vi "test_PinGroup_ReserveSessions_GroupMappingsContainsPinGroup.vi"() -> (6 "pass":bool, 8 "result":string, 15 "error out":errorcluster)   [LabVIEW 2020, in "MeasurementServerTests.lvlib" / "Session Reservation Tests.lvlib"]
uses:
  Session Reservation Tests.lvlib
  gRPC/Generated APIs/ni/measurementlink/sessionmanagement/v1/RPC Messages/ni_measurementlink_PinMapContext.ctl
  Runtime/APIs/Session Management V1/Session Reservation/Group Mapping.ctl
  Runtime/APIs/Session Management V1/Session Reservation/Session Reservation.lvclass/Session Reservation.ctl
  ab61e54b-70f9-4719-86d2-c3025959eeb5.vi
  3347d1b6-dca7-4e1a-9ca0-c9ec2f5aba95.vi
  Runtime/APIs/Session Management V1/Session Reservation/Merge Invalid DVR Error.vi
  Runtime/APIs/Session Management V1/Session Reservation/Is DVR Valid.vi
  Runtime/Measurements/Helpers/Error Strings Global Internal.vi
  <vilib>/Utility/error.llb/Error Cluster From Error Code.vi
  <vilib>/JDP Science/JSONtext/Variant to JSON Text.vi
  <vilib>/JDP Science/JSONtext/LVClass Serializer/JSONtext LVClass Serializer.lvclass
  gRPC/Generated APIs/ni/measurementlink/sessionmanagement/v1/ni.measurementlink.sessionmanagement.v1.api.lvlib
  MeasurementServerTests.lvlib
  Runtime/APIs/Session Management V1/Session Reservation/Session Reservation.lvclass
panel:
  # "Test assumes discovery service, pin map service, and session management service have already been started."
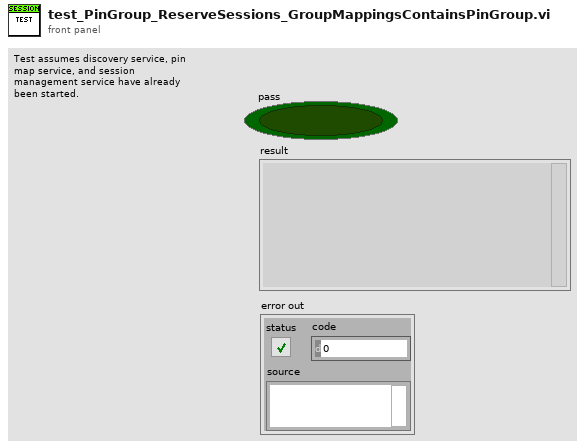
[diagram p1: front panel]
types:
  T1 = typedef "Plug-In SDK Session Management V1 API.lvlib/Session Reservation.lvclass/Group Mapping.ctl" = map{string, string[]}
  T2 = typedef "ni.measurementlink.sessionmanagement.v1.api.lvlib/ni_measurementlink_PinMapContext.ctl" = cluster{"pin_map_id":string, "sites":i32[]}
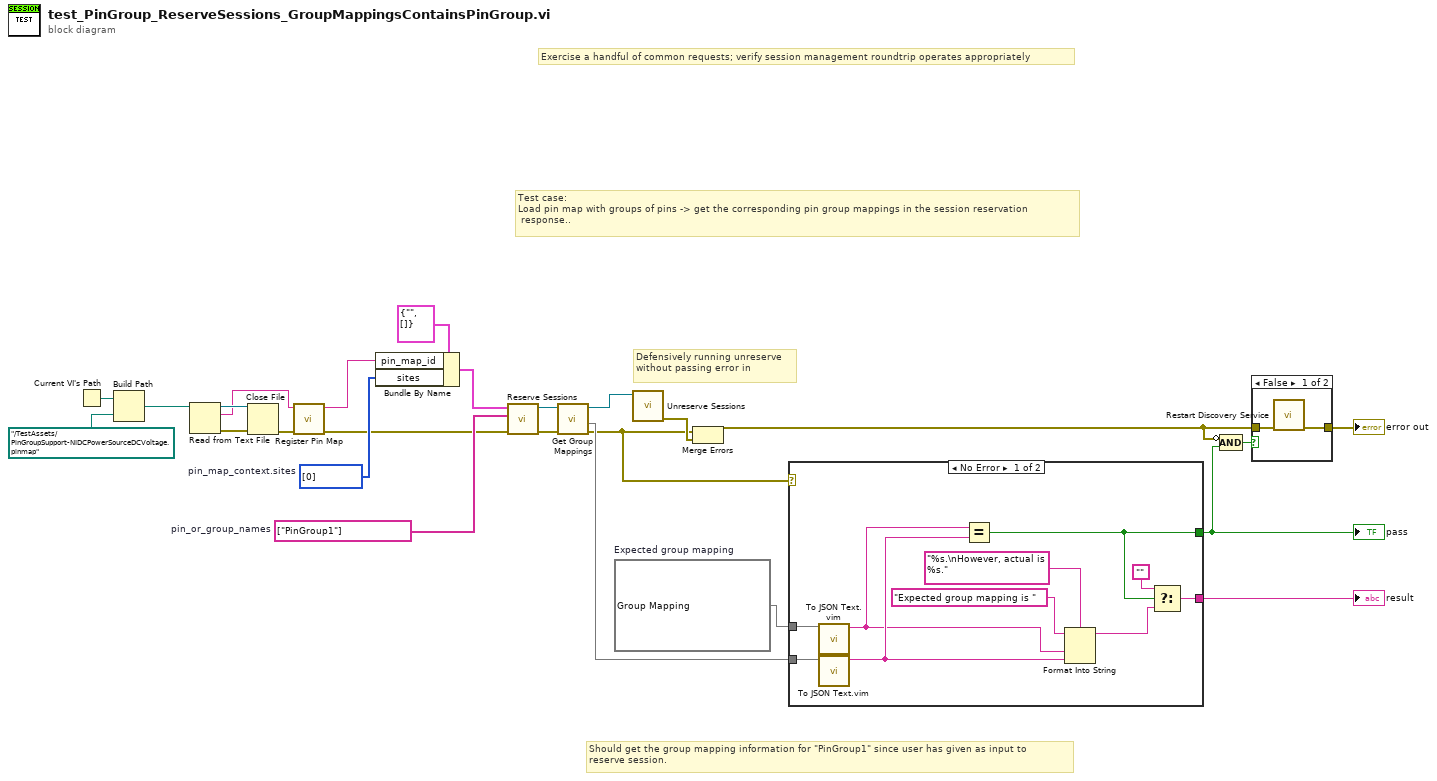
[diagram p0: block diagram]
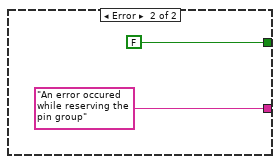
[diagram p3: hidden frame]
diagram:
  w6 = T1 {"PinGroup1"=["Pin1", "Pin2"]}  # Expected group mapping
  w15 = i32[] [0]  # pin_map_context.sites
  w12 = string[] ["PinGroup1"]  # pin_or_group_names
  # "Should get the group mapping information for \"PinGroup1\" since user has given as input to\nreserve session."
  # "Test case:\nLoad pin map with groups of pins -> get the corresponding pin group mappings in the session reservation\n\tresponse.."
  # "Defensively running unreserve without passing error in"
  # "Exercise a handful of common requests; verify session management roundtrip operates appropriately"
  n1 = Current VI's Path() -> (path=w25:path)
  n2 = Build Path(base path=w25, name or relative path=path "../TestAssets/PinGroupSupport-NIDCPowerSourceDCVoltage.pinmap") -> (appended path=w23:path)
  n3 = Read from Text File(file (use dialog)=w23) -> (refnum out=w21:refnum<file>, text=w16:string, error out=w22:errorcluster)  [unwired: 3 in, 1 out]
  n4 = Close File(refnum=w21, error in=w22) -> (error out=w17:errorcluster)  [unwired: 1 out]
  n5 = call "Register Pin Map.vi"("error in"=w17, "pin map xml"=w16) -> ("error out"=w11:errorcluster, "pin map id"=w18:string)  [unwired: 8 in]
  n6 = Bundle By Name(cluster=T2 {"pin_map_id"="", "sites"=[]} ("pin map context"), "pin_map_id"=w18, "sites"=w15) -> (w13:T2)
  n7 = call "Reserve Sessions.vi"("error in"=w11, "pin or relay names"=w12, "pin map context"=w13) -> ("error out"=w8:errorcluster, "session reservation out"=w9:refnum<class "Session Reservation.lvclass">)  [unwired: 7 in]
  n8 = call "Get Group Mappings.vi"("error in"=w8, "session reservation in"=w9) -> ("error out"=w4:errorcluster, "group mappings"=w5:T1, "session reservation out"=w7:refnum<class "Session Reservation.lvclass">)  [unwired: 7 in]
  n9 = call "Unreserve Sessions.vi"("session reservation in"=w7) -> ("error out"=w10:errorcluster)  [unwired: 10 in]
  n10 = Merge Errors(w4, w10) -> (w1:errorcluster)
  n11 = case shown="No Error" w4 {
    tunnel: [w35 FALSE] -> w3
    tunnel: [w34 "An error occured while reserving the pin group" ("String")] -> w20
    tunnel: w6 -> [w28 _]
    tunnel: w5 -> [w29 _]
    frame No Error {
      n12 = call "To JSON Text.vim"("Anything"=w28) -> ("<JSON>"=w26:string)  [unwired: 9 in, 1 out]
      n13 = call "To JSON Text.vim"("Anything"=w29) -> ("<JSON>"=w27:string)  [unwired: 9 in, 1 out]
      n14 = Equal?(x=w26, y=w27) -> (x = y?=w35:bool)
      n15 = Format Into String(format string="%s.\nHowever, actual is %s.", initial string="Expected group mapping is ", w26, w27) -> (resulting string=w30:string)  [unwired: 1 in, 1 out]
      n16 = Select(t="", s=w35, f=w30) -> (s? t:f=w34:string)
    }
    frame Error {
    }
  }
  "pass" <- w3
  "result" <- w20
  n17 = Compound Arithmetic op=AND(invert w1, w3) -> (w2:bool)
  n18 = case shown="False" w2 {
    tunnel: [w39 w40] -> w14
    tunnel: w1 -> [w38 w40]
    frame False {
      n19 = call "Restart Discovery Service.vi"("error in"=w38) -> ("error out"=w39:errorcluster)  [unwired: 10 in]
    }
    frame True {
    }
  }
  "error out" <- w14
